vi "clear connection.vi"(8 "error in (no error)":errorcluster, 11 "tcp server connection in":refnum<class "tcp server connection.lvclass">) -> (0 "error out":errorcluster, 3 "tcp server connection out":refnum<class "tcp server connection.lvclass">)   [LabVIEW 2014, in "tcp server connection.lvclass"]
doc: "This vi will execute normally even if there is an incoming error."
uses:
  tcp server connection.lvclass
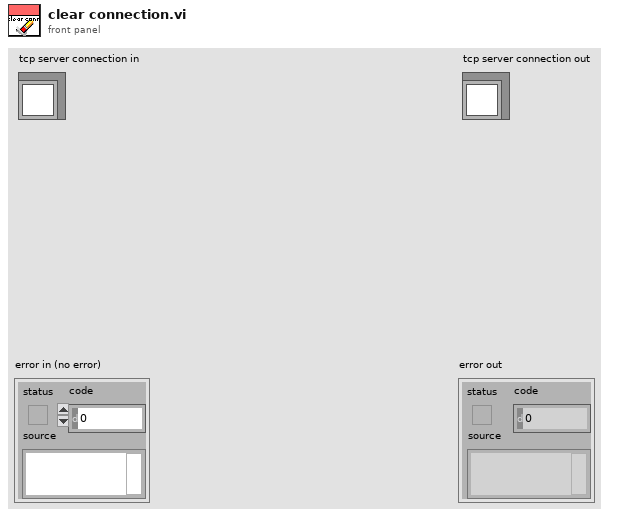
[diagram p1: front panel]
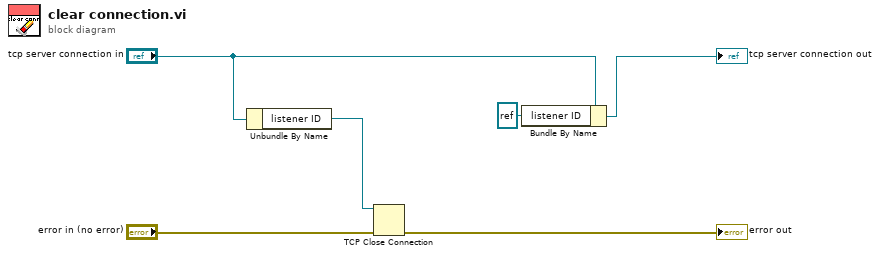
[diagram p0: block diagram]
diagram:
  n1 = Unbundle By Name("tcp server connection in") -> ("listener ID"=w2:refnum<k5>)
  n2 = TCP Close Connection(connection ID=w2, error in (no error)="error in (no error)") -> (error out=→"error out":errorcluster)  [unwired: 1 in, 1 out]
  n3 = Bundle By Name(cluster="tcp server connection in", "listener ID"=refnum<k5> refnum) -> (→"tcp server connection out":refnum<class "tcp server connection.lvclass">)
